vi "Restore Graph Property.vi"(6 "Control Ref Queue":T1, 7 "Polar?":bool, 8 "error in (no error)":errorcluster, 11 "2D Compass.lvclass in":refnum<class "2D Compass.lvclass">) -> (0 "error out":errorcluster, 3 "2D Compass.lvclass out":refnum<class "2D Compass.lvclass">)   [LabVIEW 2017, in "2D Compass.lvclass"]
uses:
  <vilib>/Math Plots/2D Math Plots/2D Compass/2D Compass/2D Compass.lvclass
  <vilib>/Math Plots/2D Math Plots/2D Plot/Action String/2DMathPlot Ctrl Act Queue.ctl
  <vilib>/Math Plots/2D Math Plots/2D Plot/Action String/2DMathPlot Ctrl Act Cluster.ctl
  <vilib>/Math Plots/2D Math Plots/2D Plot/Action String/2DMathPlot State Class.ctl
  <vilib>/Math Plots/2D Math Plots/2D Compass/2D Compass/2D Compass.lvclass/2D Compass.ctl
  <vilib>/Math Plots/2D Math Plots/2D Plot/2D Plot/2D Plot.lvclass
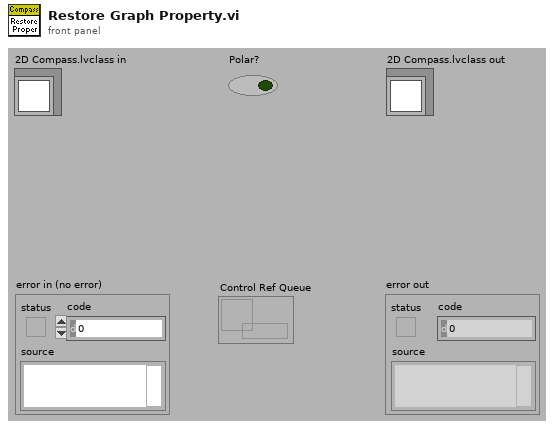
[diagram p1: front panel]
types:
  T1 = typedef "2DMathPlot Ctrl Act Queue.ctl" = refnum<queue>
  T2 = typedef "2DMathPlot Ctrl Act Cluster.ctl" = cluster{"Plot Area Ref":refnum<vi>, "Z Axis Ref":refnum<vi>, "Legend Ref":refnum<vi>, "XControl Ref":refnum<vi>, "Facade Ref":refnum<vi>, "Display State Change Class":T3}
  T3 = typedef "2DMathPlot State Class.ctl" = enum16{"Update All (Undo)", "Update General", "Update Appearance", "Update Format", "Update Scale", "Update Marker", "Update Cursor", "None"}
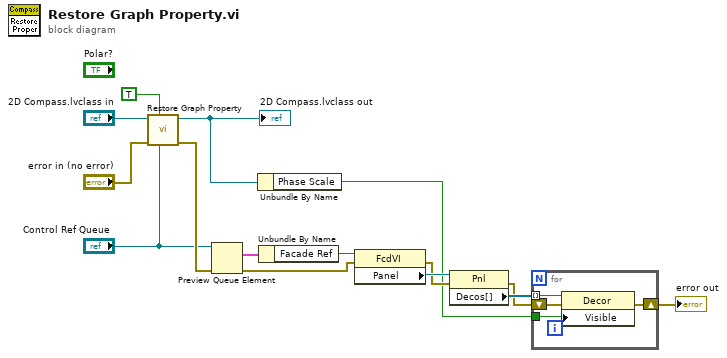
[diagram p0: block diagram]
diagram:
  n1 = call-parent "Restore Graph Property.vi"("Control Ref Queue"="Control Ref Queue", "Polor?"=TRUE, "error in (no error)"="error in (no error)", "2D Plot.lvclass in"="2D Compass.lvclass in") -> ("error out"=w3:errorcluster, "2D Plot.lvclass out"=w5:refnum<class "2D Compass.lvclass">)  [unwired: 1 in, 5 out]
  "2D Compass.lvclass out" <- w5
  n2 = Preview Queue Element(queue="Control Ref Queue", error in (no error)=w3) -> (element=w10:T2, error out=w1:errorcluster)  [unwired: 3 out]
  n3 = Unbundle By Name(w5) -> ("Phase Scale"=w11:bool)
  n4 = Unbundle By Name(w10) -> ("Facade Ref"=w9:refnum<vi>)
  n5 = property class="FcdVI"(reference=w9, error in=w1) -> (error out=w13:errorcluster, "Panel"=w15:refnum<vi>)  [unwired: 1 out]
  n6 = property class="Pnl"(reference=w15, error in=w13) -> (error out=w12:errorcluster, "Decos[]"=w14:refnum<vi>[])  [unwired: 1 out]
  n7 = for {
    tunnel: w14 -> [w19] mode=indexing
    tunnel: w11 -> [w18]
    shift-right: [w16] -> w8
    shift-left: w12 -> [w17]
    n8 = property class="Decor"(reference=w19, error in=w17, "Visible"=w18) -> (error out=w16:errorcluster)  [unwired: 1 out]
  }
  "error out" <- w8
